vi "CharToHex.vi"(11 "Character":string) -> (3 "Hex":i32 format="%x")   [LabVIEW 2018]
uses:
  <vilib>/regexp/Match Regular Expression.xnode
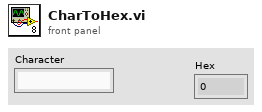
[diagram p1: front panel]
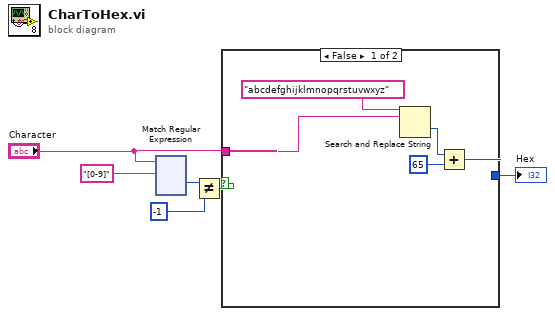
[diagram p0: block diagram]
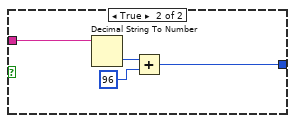
[diagram p2: hidden frame]
diagram:
  n1 = xnode "Match Regular Expression"("input string"="Character", "regular expression"="[0-9]") -> ("offset past match"=w5:i32)  [unwired: 4 in, 4 out]
  n2 = Not Equal?(x=w5, y=-1) -> (x != y?=w3:bool)
  n3 = case shown="False" w3 {
    tunnel: "Character" -> [w11 w15]
    tunnel: [w8 w12] -> w1
    frame False {
      n4 = Search and Replace String(input string="abcdefghijklmnopqrstuvwxyz", search string=w11) -> (offset past replacement=w7:i32)  [unwired: 6 in, 3 out]
      n5 = Add(x=w7, y=65) -> (x+y=w8:i32)
    }
    frame True {
      n6 = Decimal String To Number(string=w15) -> (number=w14:i32)  [unwired: 2 in, 1 out]
      n7 = Add(x=w14, y=96) -> (x+y=w12:i32)
    }
  }
  "Hex" <- w1
